vi "Log Error File.vi"(8 "error in (no error)":errorcluster, 11 "Log String":string) -> (0 "error out":errorcluster)   [LabVIEW 2017]
doc: "Author: Scott Hannahs <sth@magnet.fsu.edu>\nCopyright 2018 Florida State University, All rights reserved."
uses:
  <vilib>/Utility/error.llb/DialogType.ctl
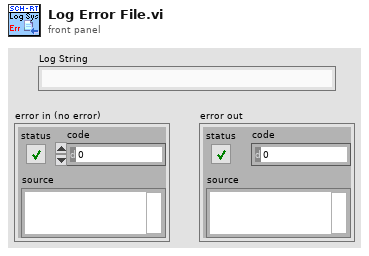
[diagram p1: front panel]
types:
  T1 = typedef "DialogType.ctl" = u16
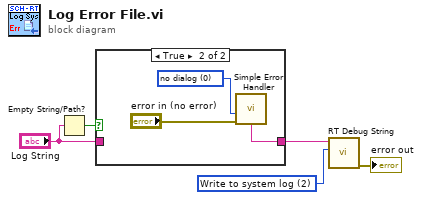
[diagram p0: block diagram]
diagram:
  w3 = u16 2 items=["Write to serial", "Write to monitor", "Write to system log"] ("Interface")
  n1 = Empty String/Path?(string/path="Log String") -> (empty?=w2:bool)
  n2 = case shown="True" w2 {
    tunnel: [w6 w8] -> w4
    tunnel: "Log String" -> [w6 _]
    frame False {
    }
    frame True {
      w7 = T1 0 items=["no dialog", "OK message", "continue or stop message", "OK message + warnings", "continue/stop + warnings"] ("type of dialog (OK msg:1)")
      n3 = call <vilib>:"Simple Error Handler.vi"("type of dialog (OK msg:1)"=w7, "error in (no error)"="error in (no error)") -> ("message"=w8:string)  [unwired: 3 in, 4 out]
    }
  }
  n4 = call <vilib>:"RT Debug String.vi"("Interface"=w3, "String to write"=w4) -> ("error out"=→"error out":errorcluster)  [unwired: 9 in]
